vi "ToString.vi"(8 "error in (no error)":errorcluster, 11 "Collection Is Empty in":refnum<class "Collection Is Empty.lvclass">) -> (0 "error out":errorcluster, 2 "String":string, 3 "Collection Is Empty out":refnum<class "Collection Is Empty.lvclass">)   [LabVIEW 2017, in "Transparent Assertions.lvlib" / "Collection Is Empty.lvclass"]
doc: "Returns a string representation of the object."
uses:
  Collection Is Empty.lvclass
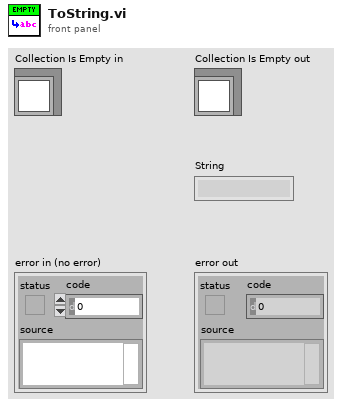
[diagram p1: front panel]
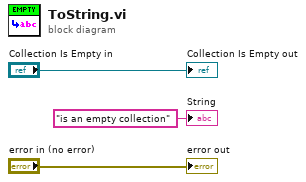
[diagram p0: block diagram]
diagram:
  "error out" <- "error in (no error)"
  "Collection Is Empty out" <- "Collection Is Empty in"
  "String" <- "is an empty collection" ("String")
